vi "Exemple_Metrics_Pairwise_Distances_Chunked.vi"() -> ()   [LabVIEW 2020]
uses:
  Objet/6 - Datasets Transformation/6.8 - Pairwise metrics, Affinities and Kernels/Pairwise_distances_chunked/Pairwise_distances_chunked.vi
panel:
  in  "pairwise_distances_chunked":T1={"reduce_func"="None", "metric "="euclidean", "n_jobs"="None", "working_memory"="None"}
  in  "error in":errorcluster caption="entrée d'erreur"
  in  "Y":string[][](array[string])=[["1", "0"], ["2", "1"]]
  in  "X":string[][](array[string])=[["2", "3"], ["3", "5"], ["5", "8"]]
  out "Data":T2
  out "error out":errorcluster caption="sortie d'erreur"
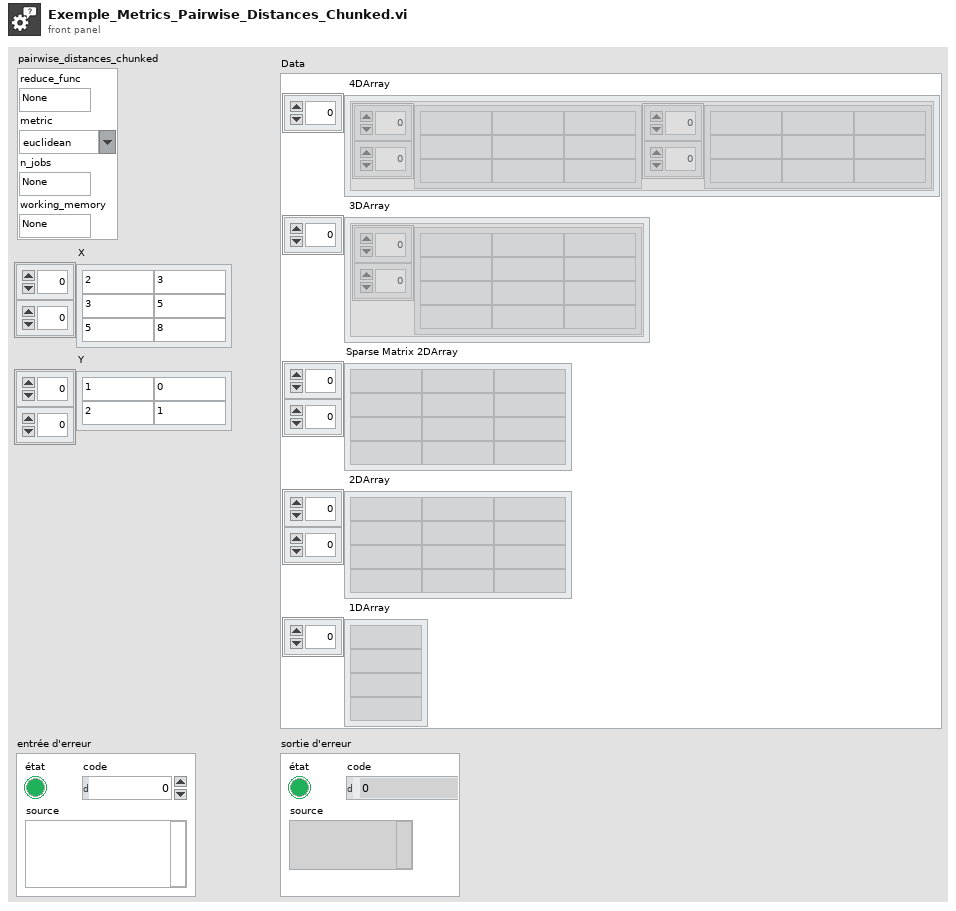
[diagram p1: front panel]
types:
  T1 = cluster{"reduce_func":string, "metric ":string, "n_jobs":string, "working_memory":string}
  T2 = cluster{" 4DArray":cluster{"1":string[][], "2":string[][]}[], " 3DArray":cluster{"Tableau":string[][]}[], "Sparse Matrix 2DArray":string[][], " 2DArray":string[][], " 1DArray":string[]}
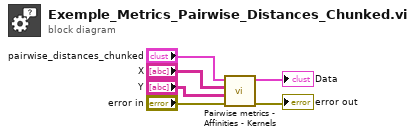
[diagram p0: block diagram]
diagram:
  n1 = call-poly "Pairwise metrics - Affinities - Kernels.vi"("error in"="error in", "Y"="Y", "X"="X", "pairwise_distances_chunked"="pairwise_distances_chunked") -> ("error out"=→"error out":errorcluster, "Data"=→"Data":T2)  [unwired: 6 in]
